vi "poly_h5_write_array_3d_DBL.vi"(0 "h5 dir ref":i32, 1 "dataset name":string, 5 "3d array":dbl[][][](array[numeric]), 7 "units (au)":string="au", 11 "error in (no error)":errorcluster, 12 "dim1 (index)":string="index", 13 "dim2 (index)":string="index", 14 "dim3 (index)":string="index") -> (4 "h5 obj ref":i32, 15 "error out":errorcluster)   [LabVIEW 2015]
uses:
  <vilib>/addons/h5labview2/base/lib_path.vi
  <vilib>/addons/h5labview2/base/H5Equery.vi
  <vilib>/addons/h5labview2/dataset/H5Dwrite.llb/H5Dwrite.xnode
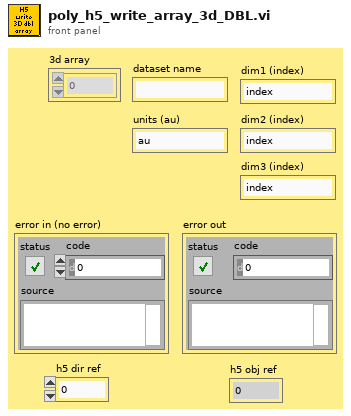
[diagram p1: front panel]
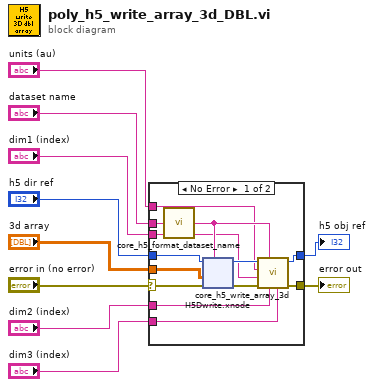
[diagram p0: block diagram]
diagram:
  n1 = case shown="No Error" "error in (no error)" {
    selector: "error in (no error)" -> [w21 w44]
    tunnel: "h5 dir ref" -> [w23 w43]
    tunnel: "3d array" -> [w22 _]
    tunnel: [w16 w44] -> w8
    tunnel: [w19 w43] -> w7
    tunnel: "dataset name" -> [w18 _]
    tunnel: "units (au)" -> [w14 _]
    tunnel: "dim2 (index)" -> [w13 _]
    tunnel: "dim3 (index)" -> [w12 _]
    tunnel: "dim1 (index)" -> [w11 _]
    frame No Error {
      n2 = call "core_h5_format_dataset_name.vi"("dataset name in"=w18) -> ("dataset name out"=w15:string)  [unwired: 8 in]
      n3 = xnode "H5Dwrite.xnode"("dataset name"=w15, "error in (no error)"=w21, "data"=w22, "ref in"=w23) -> ("error out"=w17:errorcluster, "ref out"=w20:i32)  [unwired: 3 in, 1 out]
      n4 = call "core_h5_write_array_3d.vi"("dim3 (index)"=w12, "dim2 (index)"=w13, "dataset name"=w15, "error in (no error)"=w17, "dim1 (index)"=w11, "units (au)"=w14, "h5 obj ref"=w20) -> ("error out"=w16:errorcluster, "h5 obj ref"=w19:i32)  [unwired: 3 in]
    }
    frame Error {
    }
  }
  "error out" <- w8
  "h5 obj ref" <- w7
